vi "ReadSubVI.vi"(1 "reference":refnum<vi>) -> (0 "SubVI":T5)   [LabVIEW 2013]
uses:
  <vilib>/Utility/miscctls.llb/LVBoundsTypeDef.ctl
  <vilib>/Utility/miscctls.llb/LVPositionTypeDef.ctl
  <vilib>/Utility/miscctls.llb/LVRectTypeDef.ctl
  <vilib>/Utility/miscctls.llb/LVBreakpointStatusEnum.ctl
panel:
  out "error out 31":errorcluster
  out "error out 30":errorcluster
  out "error out 29":errorcluster
  out "error out 28":errorcluster
  out "error out 27":errorcluster
  out "error out 26":errorcluster
  out "error out 25":errorcluster
  out "error out 24":errorcluster
  out "error out 23":errorcluster
  out "error out 22":errorcluster
  out "error out 21":errorcluster
  out "error out 20":errorcluster
  out "error out 19":errorcluster
  out "error out 18":errorcluster
  out "error out 17":errorcluster
  out "error out 16":errorcluster
  out "error out 15":errorcluster
  out "error out 14":errorcluster
  out "error out 13":errorcluster
  out "error out 12":errorcluster
  out "error out 11":errorcluster
  out "error out 10":errorcluster
  out "error out 9":errorcluster
  out "error out 8":errorcluster
  out "error out 7":errorcluster
  out "error out 6":errorcluster
  out "error out 5":errorcluster
  out "error out 4":errorcluster
  out "error out 3":errorcluster
  out "error out 2":errorcluster
  out "error out":errorcluster
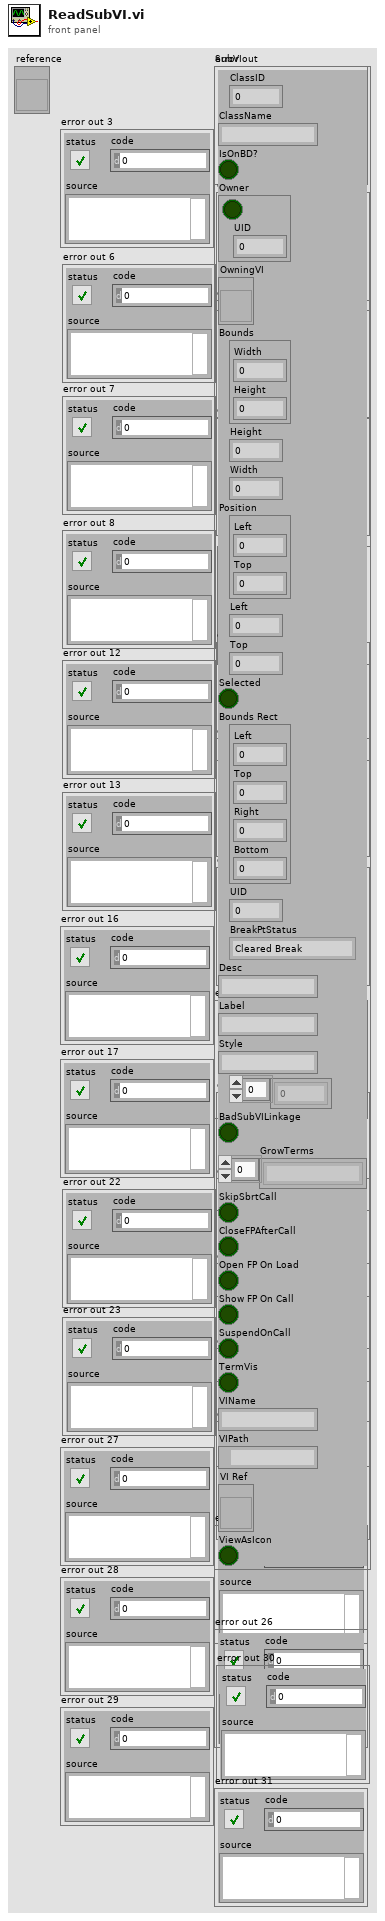
[diagram p1: front panel]
types:
  T1 = typedef "LVBoundsTypeDef.ctl" = cluster{"Width":u32, "Height":u32}
  T2 = typedef "LVPositionTypeDef.ctl" = cluster{"Left":i32, "Top":i32}
  T3 = typedef "LVRectTypeDef.ctl" = cluster{"Left":i16, "Top":i16, "Right":i16, "Bottom":i16}
  T4 = typedef "LVBreakpointStatusEnum.ctl" = enum8{"Cleared Break", "Enabled Break", "Disabled Break"}
  T5 = cluster{"ClassID":u32, "ClassName":string, "IsOnBD?":bool, "Owner":cluster{bool, "UID":i32}, "OwningVI":refnum<vi>, "Bounds":T1, "Height":u32, "Width":u32, "Position":T2, "Left":i32, "Top":i32, "Selected":bool, "Bounds Rect":T3, "UID":i32, "BreakPtStatus":T4, "Desc":string, "Label":string, "Style":string, "Terms[]":i32[], "BadSubVILinkage":bool, "GrowTerms":string[], "SkipSbrtCall":bool, "CloseFPAfterCall":bool, "Open FP On Load":bool, "Show FP On Call":bool, "SuspendOnCall":bool, "TermVis":bool, "VIName":string, "VIPath":path, "VI Ref":refnum<vi>, "ViewAsIcon":bool}
  T6 = cluster{"ClassID":u32, "ClassName":string, "IsOnBD?":bool, "Cluster":cluster{bool, "UID":i32}, "OwningVI":refnum<vi>, "Bounds":T1, "Height":u32, "Width":u32, "Position":T2, "Left":i32, "Top":i32, "Selected":bool, "Bounds Rect":T3, "UID":i32, "BreakPtStatus":T4, "Desc":string, "Text":string, "Style":string, i32[], "BadSubVILinkage":bool, "GrowTerms":string[], "SkipSbrtCall":bool, "CloseFPAfterCall":bool, "Open FP On Load":bool, "Show FP On Call":bool, "SuspendOnCall":bool, "TermVis":bool, "VIName":string, "VIPath":path, "VI Ref":refnum<vi>, "ViewAsIcon":bool}
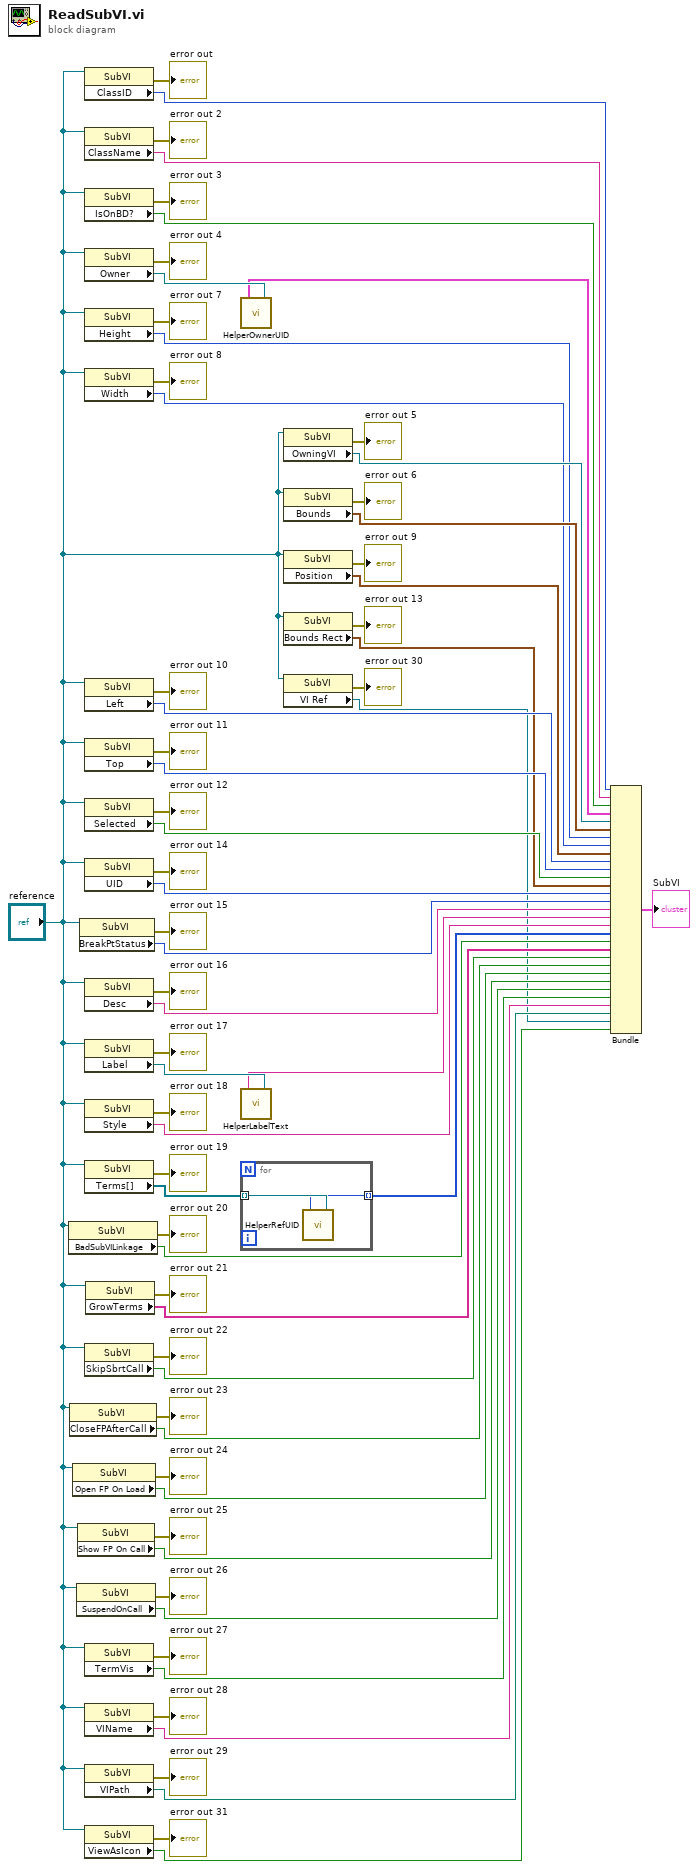
[diagram p0: block diagram]
diagram:
  n1 = property class="SubVI"(reference="reference") -> (error out=→"error out 20":errorcluster, "BadSubVILinkage"=w24:bool)  [unwired: 1 in, 1 out]
  n2 = property class="SubVI"(reference="reference") -> (error out=→"error out 23":errorcluster, "CloseFPAfterCall"=w18:bool)  [unwired: 1 in, 1 out]
  n3 = property class="SubVI"(reference="reference") -> (error out=→"error out 24":errorcluster, "Open FP On Load"=w16:bool)  [unwired: 1 in, 1 out]
  n4 = property class="SubVI"(reference="reference") -> (error out=→"error out 26":errorcluster, "SuspendOnCall"=w12:bool)  [unwired: 1 in, 1 out]
  n5 = property class="SubVI"(reference="reference") -> (error out=→"error out 25":errorcluster, "Show FP On Call"=w14:bool)  [unwired: 1 in, 1 out]
  n6 = property class="SubVI"(reference="reference") -> (error out=→"error out 15":errorcluster, "BreakPtStatus"=w36:T4)  [unwired: 1 in, 1 out]
  n7 = property class="SubVI"(reference="reference") -> (error out=→"error out":errorcluster, "ClassID"=w65:u32)  [unwired: 1 in, 1 out]
  n8 = property class="SubVI"(reference="reference") -> (error out=→"error out 2":errorcluster, "ClassName"=w63:string)  [unwired: 1 in, 1 out]
  n9 = property class="SubVI"(reference="reference") -> (error out=→"error out 3":errorcluster, "IsOnBD?"=w61:bool)  [unwired: 1 in, 1 out]
  n10 = property class="SubVI"(reference="reference") -> (error out=→"error out 4":errorcluster, "Owner"=w59:refnum<vi>)  [unwired: 1 in, 1 out]
  n11 = property class="SubVI"(reference="reference") -> (error out=→"error out 7":errorcluster, "Height"=w52:u32)  [unwired: 1 in, 1 out]
  n12 = property class="SubVI"(reference="reference") -> (error out=→"error out 8":errorcluster, "Width"=w50:u32)  [unwired: 1 in, 1 out]
  n13 = property class="SubVI"(reference="reference") -> (error out=→"error out 10":errorcluster, "Left"=w46:i32)  [unwired: 1 in, 1 out]
  n14 = property class="SubVI"(reference="reference") -> (error out=→"error out 11":errorcluster, "Top"=w44:i32)  [unwired: 1 in, 1 out]
  n15 = property class="SubVI"(reference="reference") -> (error out=→"error out 12":errorcluster, "Selected"=w42:bool)  [unwired: 1 in, 1 out]
  n16 = property class="SubVI"(reference="reference") -> (error out=→"error out 14":errorcluster, "UID"=w38:i32)  [unwired: 1 in, 1 out]
  n17 = property class="SubVI"(reference="reference") -> (error out=→"error out 16":errorcluster, "Desc"=w34:string)  [unwired: 1 in, 1 out]
  n18 = property class="SubVI"(reference="reference") -> (error out=→"error out 17":errorcluster, "Label"=w32:refnum<vi>)  [unwired: 1 in, 1 out]
  n19 = property class="SubVI"(reference="reference") -> (error out=→"error out 18":errorcluster, "Style"=w29:string)  [unwired: 1 in, 1 out]
  n20 = property class="SubVI"(reference="reference") -> (error out=→"error out 19":errorcluster, "Terms[]"=w27:refnum<vi>[])  [unwired: 1 in, 1 out]
  n21 = property class="SubVI"(reference="reference") -> (error out=→"error out 22":errorcluster, "SkipSbrtCall"=w20:bool)  [unwired: 1 in, 1 out]
  n22 = property class="SubVI"(reference="reference") -> (error out=→"error out 27":errorcluster, "TermVis"=w10:bool)  [unwired: 1 in, 1 out]
  n23 = property class="SubVI"(reference="reference") -> (error out=→"error out 28":errorcluster, "VIName"=w8:string)  [unwired: 1 in, 1 out]
  n24 = property class="SubVI"(reference="reference") -> (error out=→"error out 29":errorcluster, "VIPath"=w6:path)  [unwired: 1 in, 1 out]
  n25 = property class="SubVI"(reference="reference") -> (error out=→"error out 31":errorcluster, "ViewAsIcon"=w2:bool)  [unwired: 1 in, 1 out]
  n26 = property class="SubVI"(reference="reference") -> (error out=→"error out 21":errorcluster, "GrowTerms"=w22:string[])  [unwired: 1 in, 1 out]
  n27 = call "HelperOwnerUID.vi"("Generic in"=w59) -> ("Cluster"=w58:cluster{bool, "UID":i32})
  n28 = call "HelperLabelText.vi"("Text in"=w32) -> ("Text"=w31:string)
  n29 = for {
    tunnel: w27 -> [w69] mode=indexing
    tunnel: [w68] -> w26 mode=indexing
    n30 = call "HelperRefUID.vi"("Text in"=w69) -> ("UID"=w68:i32)
  }
  n31 = property class="SubVI"(reference="reference") -> (error out=→"error out 5":errorcluster, "OwningVI"=w56:refnum<vi>)  [unwired: 1 in, 1 out]
  n32 = property class="SubVI"(reference="reference") -> (error out=→"error out 6":errorcluster, "Bounds"=w54:T1)  [unwired: 1 in, 1 out]
  n33 = property class="SubVI"(reference="reference") -> (error out=→"error out 9":errorcluster, "Position"=w48:T2)  [unwired: 1 in, 1 out]
  n34 = property class="SubVI"(reference="reference") -> (error out=→"error out 13":errorcluster, "Bounds Rect"=w40:T3)  [unwired: 1 in, 1 out]
  n35 = property class="SubVI"(reference="reference") -> (error out=→"error out 30":errorcluster, "VI Ref"=w4:refnum<vi>)  [unwired: 1 in, 1 out]
  n36 = Bundle("ClassID"=w65, "ClassName"=w63, "IsOnBD?"=w61, "Cluster"=w58, "OwningVI"=w56, "Bounds"=w54, "Height"=w52, "Width"=w50, "Position"=w48, "Left"=w46, "Top"=w44, "Selected"=w42, "Bounds Rect"=w40, "UID"=w38, "BreakPtStatus"=w36, "Desc"=w34, "Text"=w31, "Style"=w29, w26, "BadSubVILinkage"=w24, "GrowTerms"=w22, "SkipSbrtCall"=w20, "CloseFPAfterCall"=w18, "Open FP On Load"=w16, "Show FP On Call"=w14, "SuspendOnCall"=w12, "TermVis"=w10, "VIName"=w8, "VIPath"=w6, "VI Ref"=w4, "ViewAsIcon"=w2) -> (→"SubVI":T6)  [unwired: 1 in]
